vi "Algae Teleop Handler.vi"() -> ()   [LabVIEW 2023]
uses:
  Teleop Util/Algae States.ctl
  <vilib>/Rock Robotics/WPI/Joystick/XBox Buttons Indexer.ctl
  <vilib>/Rock Robotics/WPI/Joystick/XBox Axes Indexer.ctl
  Algae/Implementation/Algae Operations.ctl
  918af4a3-8dae-4537-8dc6-29252aaed449.vi
  <vilib>/Rock Robotics/WPI/Utilities/WPI_GetSetVariantRefNum.vi
  Framework/Robot Global Data.vi
panel:
  in  "Setpoint":dbl
  out "s? t:f":T1=enum."Intake Algae"
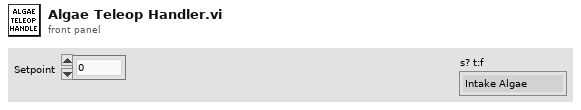
[diagram p1: front panel]
types:
  T1 = typedef "Algae States.ctl" = enum16{"Idle", "Intake Algae", "Outtake Algae", "Stow", "Manual Overrides", "Fling"}
  T2 = typedef "XBox Axes Indexer.ctl" = enum16{"Left X", "Left Y", "Left Trigger", "Right Trigger", "Right X", "Right Y"}
  T3 = typedef "XBox Buttons Indexer.ctl" = enum16{"A", "B", "X", "Y", "Left Bumper", "Right Bumper", "Back", "Start", "Left Joystick", "Right Joystick"}
  T4 = typedef "WPI_JoystickDevRef.ctl" = cluster{"Device":T5}
  T5 = typedef "WPI_JoystickDeviceEnum.ctl" = enum16{"USB 0", "USB 1", "USB 2", "USB 3", "USB 4", "USB 5"}
  T6 = typedef "Algae Operations.ctl" = enum16{"Reserve", "Read Current", "Immediate", "Calibrate"}
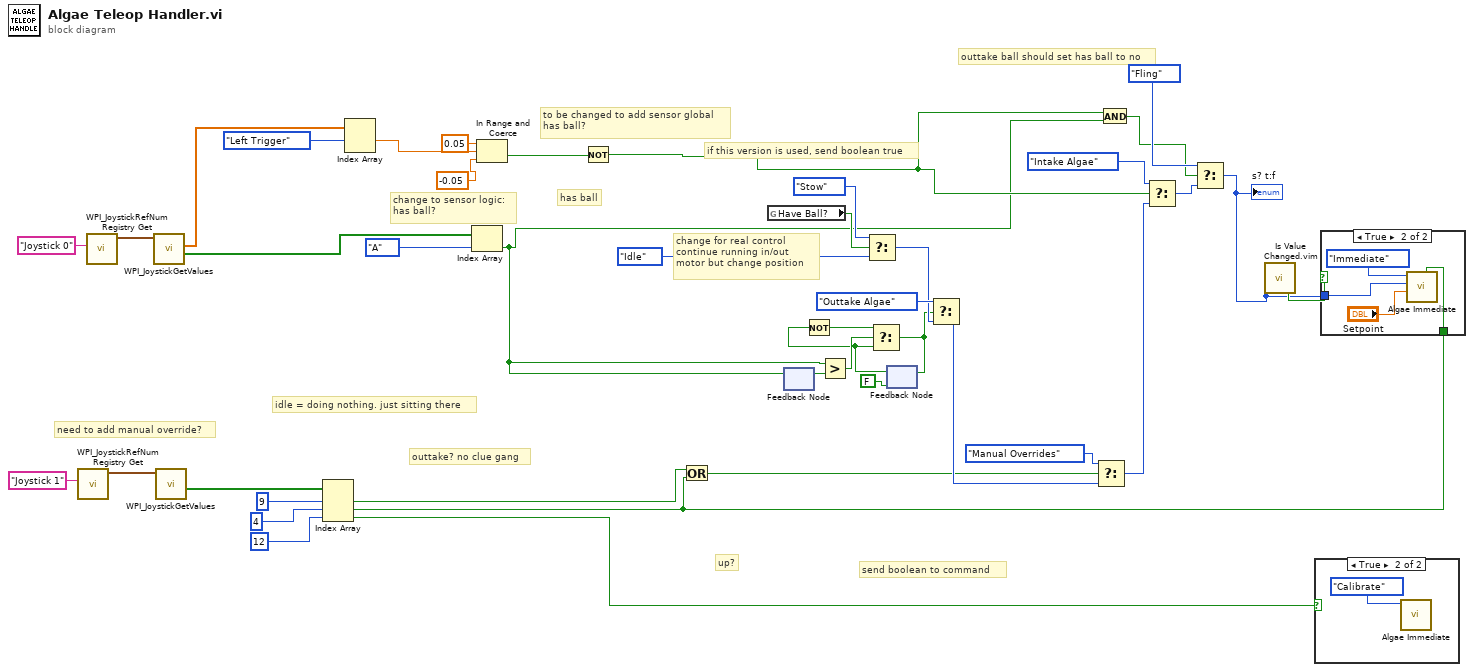
[diagram p0: block diagram]
diagram:
  # "send boolean to command"
  # "up?"
  # "if this version is used, send boolean true"
  # "outtake? no clue gang"
  # "outtake ball should set has ball to no"
  # "has ball"
  # "change for real control\ncontinue running in/out\nmotor but change position"
  # "to be changed to add sensor global\nhas ball?"
  # "need to add manual override?"
  # "idle = doing nothing. just sitting there"
  # "change to sensor logic:\nhas ball?"
  n1 = call <vilib>:"WPI_JoystickRefNum Registry Get.vi"("refnum name"="Joystick 1") -> ("JoystickDevRef"=w30:T4)  [unwired: 1 in, 9 out]
  n2 = call <vilib>:"WPI_JoystickRefNum Registry Get.vi"("refnum name"="Joystick 0") -> ("JoystickDevRef"=w41:T4)  [unwired: 1 in, 9 out]
  n3 = call <vilib>:"WPI_JoystickGetValues.vi"("JoystickDevRef"=w41) -> ("Buttons"=w40:bool[], "Axes"=w35:dbl[])  [unwired: 6 in, 3 out]
  n4 = call <vilib>:"WPI_JoystickGetValues.vi"("JoystickDevRef"=w30) -> ("Buttons"=w24:bool[])  [unwired: 6 in, 4 out]
  n5 = Index Array(array=w24, index #1=9 ("index"), index #2=4 ("index"), index #3=12 ("index")) -> (element #1=w17:bool, element #2=w16:bool, element #3=w23:bool)
  n6 = Index Array(array=w35, index #1=XBox_Axes_Indexer."Left Trigger" ("XBox Axes")) -> (element #1=w34:dbl)  [unwired: 1 in, 1 out]
  n7 = Index Array(array=w40, index=XBox_Buttons_Indexer."A" ("XBox Buttons")) -> (element=w2:bool)
  n8 = In Range and Coerce(upper limit=0.05 ("lower limit"), x=w34, lower limit=-0.05) -> (In Range?=w36:bool)  [unwired: 1 out]
  n9 = Not(x=w36) -> (.not. x?=w3:bool)
  n10 = Or(x=w17, y=w16) -> (x .or. y?=w18:bool)
  n11 = global read "Robot Global Data.vi" "Have Ball?"() -> (w19:bool)
  n12 = feedback-in #1(w2) -> ()
  n13 = feedback #1() -> (w12:bool)  [unwired: 1 in]
  n14 = Greater?(x=w2, y=w12) -> (0:w11:bool)
  n15 = Select(t=Algae_States."Stow" ("f"), s=w19, f=Algae_States."Idle") -> (s? t:f=w20:T1)
  n16 = feedback #2(FALSE) -> (w9:bool)
  n17 = Not(x=w9) -> (.not. x?=w10:bool)
  n18 = Select(t=w10, s=w11, f=w9) -> (s? t:f=w7:bool)
  n19 = feedback-in #2(w7) -> ()
  n20 = Select(t=Algae_States."Outtake Algae", s=w7, f=w20) -> (s? t:f=w26:T1)
  n21 = Select(t=Algae_States."Manual Overrides", s=w18, f=w26) -> (s? t:f=w27:T1)
  n22 = And(x=w3, y=w2) -> (x .and. y?=w4:bool)
  n23 = Select(t=Algae_States."Intake Algae", s=w3, f=w27) -> (s? t:f=w6:T1)
  n24 = Select(t=Algae_States."Fling", s=w4, f=w6) -> (s? t:f=w1:T1)
  "s? t:f" <- w1
  n25 = call "Is Value Changed.vim"("value"=w1) -> ("changed or first call?"=w25:bool)
  n26 = case shown="True" w23 {
    frame False {
    }
    frame True {
      n27 = call "Algae Immediate.vi"("Operation"=Algae_Operations."Calibrate") -> ()  [unwired: 9 in, 1 out]
    }
  }
  n28 = case shown="True" w25 {
    tunnel: w1 -> [_ w46]
    tunnel: w16 -> [_ w45]
    frame False {
    }
    frame True {
      n29 = call "Algae Immediate.vi"("Operation"=Algae_Operations."Immediate", "Algae State"=w46, "Setpoint"="Setpoint", "Negate or Confirm?"=w45) -> ()  [unwired: 6 in, 1 out]
    }
  }
